vi "Write Pulse Configuration.vi"(8 "error in (no error)":errorcluster, 10 "Configuration":T1={"Pre-trigger duration"=0.01, "Post-trigger duration"=0.1, "Rate"=1000000.0, "Ranges"=[10.0], "Re-name channels"=[], "Active channels"="0:1", "External clock"=FALSE} {"Rate" format="%#_8pHz"; "Post-trigger duration" format="%#_6ps"; "Pre-trigger duration" format="%#_6ps"; "Ranges" format="%#_6pV"}, 11 "Pulse Driver in":refnum<class "Pulse Driver.lvclass">) -> (0 "error out":errorcluster, 3 "Pulse Driver out":refnum<class "Pulse Driver.lvclass">)   [LabVIEW 2019, in "Pulse Driver.lvclass"]
uses:
  Pulse Driver.lvclass
  Pusle Driver Configuration.ctl
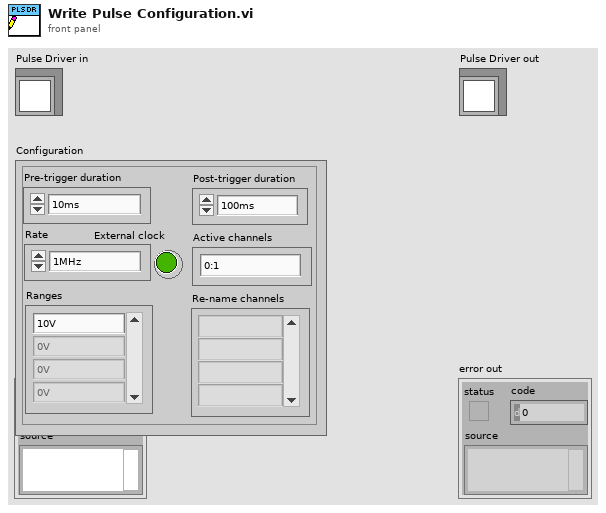
[diagram p1: front panel]
types:
  T1 = typedef "Pusle Driver Configuration.ctl" = cluster{"Pre-trigger duration":dbl, "Post-trigger duration":dbl, "Rate":dbl, "Ranges":dbl[], "Re-name channels":string[], "Active channels":string, "External clock":bool}
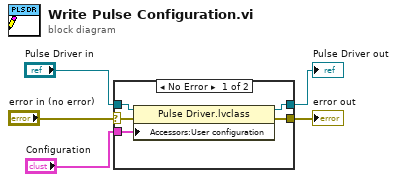
[diagram p0: block diagram]
diagram:
  n1 = case shown="No Error" "error in (no error)" {
    selector: "error in (no error)" -> [w7 w11]
    tunnel: [w6 w11] -> w4
    tunnel: [w9 w12] -> w2
    tunnel: "Pulse Driver in" -> [w10 w12]
    tunnel: "Configuration" -> [w8 _]
    frame No Error {
      n2 = property class="Pulse Driver.lvclass"(reference=w10, error in=w7, "Accessors:User configuration"=w8) -> (reference out=w9:refnum<class "Pulse Driver.lvclass">, error out=w6:errorcluster)
    }
    frame Error {
    }
  }
  "error out" <- w4
  "Pulse Driver out" <- w2
